vi "shift marks (SubVI).vi"(8 "error in (no error)":errorcluster, 9 "y":sgl, 10 "x":sgl, 11 "Application in":refnum<vi>) -> (0 "error out":errorcluster, 3 "Application out":refnum<vi>)   [LabVIEW 2014]
uses:
  <userlib>/Nanonis Prog Interface V5/Nanonis Prog Interface.lvlib
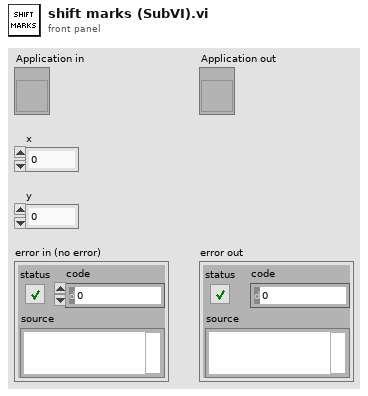
[diagram p1: front panel]
types:
  T1 = cluster{"X (m)":sgl, "Y (m)":sgl, "Text":string, "Color":u32, "Visible":bool}[]
  T2 = cluster{"x(m)":sgl, "y(m)":sgl, "Text":string, "Color":u32}
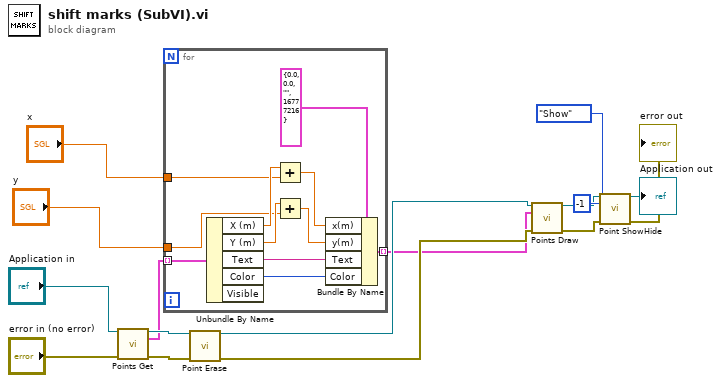
[diagram p0: block diagram]
diagram:
  n1 = call <userlib>:"Points Get.vi"("Application ref in"="Application in", "error in (no error)"="error in (no error)") -> ("Application ref out"=w7:refnum<vi>, "Points"=w2:T1, "error out"=w4:errorcluster)  [unwired: 11 in]
  n2 = for {
    tunnel: w2 -> [w23] mode=indexing
    tunnel: "x" -> [w25]
    tunnel: "y" -> [w24]
    tunnel: [w17] -> w8 mode=indexing
    n3 = Unbundle By Name(w23) -> ("X (m)"=w27:sgl, "Y (m)"=w26:sgl, "Text"=w19:string, "Color"=w18:u32)  [unwired: 1 out]
    n4 = Add(x=w27, y=w25) -> (x+y=w21:sgl)
    n5 = Add(x=w26, y=w24) -> (x+y=w20:sgl)
    n6 = Bundle By Name(cluster=T2 {"x(m)"=0.0, "y(m)"=0.0, "Text"="", "Color"=16777216} ("Point"), "x(m)"=w21, "y(m)"=w20, "Text"=w19, "Color"=w18) -> (w17:T2)
  }
  n7 = call <userlib>:"Point Erase.vi"("Application ref in"=w7, "error in (no error)"=w4) -> ("Application ref out"=w14:refnum<vi>, "error out"=w13:errorcluster)  [unwired: 12 in]
  n8 = call <userlib>:"Points Draw.vi"("Application ref in"=w14, "Points Configuration"=w8, "error in (no error)"=w13) -> ("Application ref out"=w9:refnum<vi>, "error out"=w12:errorcluster)  [unwired: 11 in]
  n9 = call <userlib>:"Point ShowHide.vi"("Application ref in"=w9, "Point index (-1=All points)"=-1, "Show/Hide"=enum16{"Show", "Hide"}."Show", "error in (no error)"=w12) -> ("Application ref out"=→"Application out":refnum<vi>, "error out"=→"error out":errorcluster)  [unwired: 10 in]
